vi "HX_Water-Props.vi"(8 "error in (no error)":errorcluster, 11 "Water Avg (°F)":dbl) -> (0 "error out":errorcluster, 2 "mu (lbm/ft*s)":dbl, 3 "Cp (BTU/lbm°F)":dbl, 4 "Density (lbm/ft³)":dbl)   [LabVIEW 2012]
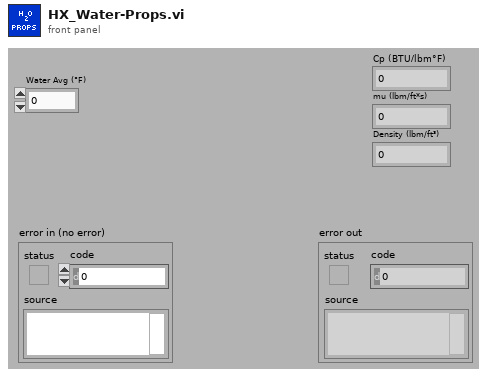
[diagram p1: front panel]
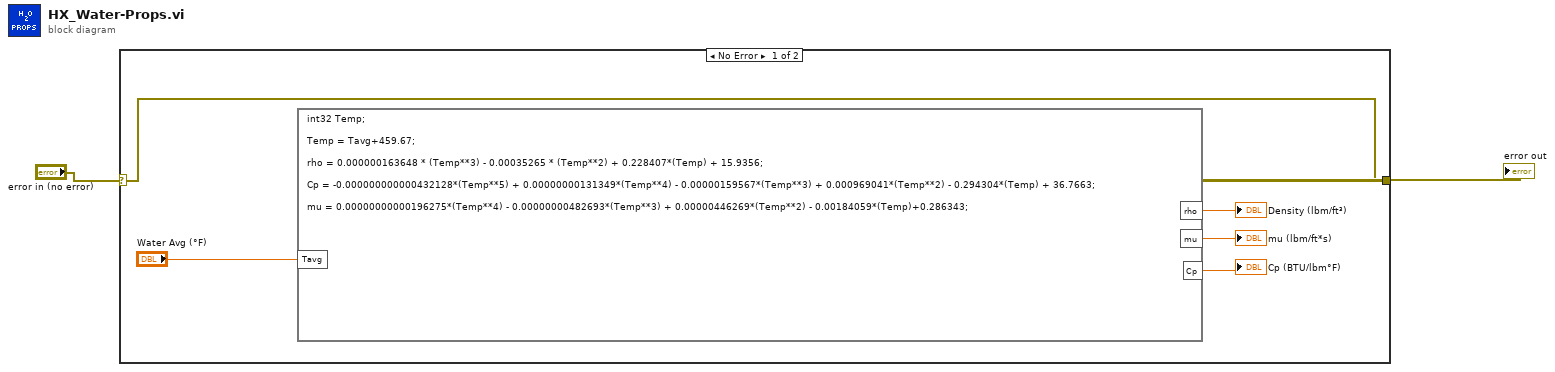
[diagram p0: block diagram]
diagram:
  n1 = case shown="No Error" "error in (no error)" {
    selector: "error in (no error)" -> [w3 w8]
    tunnel: [w3 w8] -> w1
    frame No Error {
      n2 = formula code="int32 Temp;\n \nTemp = Tavg+459.67;\n\nrho = 0.000000163648 * (Temp**3) - 0.00035265 * (Temp**2) + 0.228407*(Temp) + 15.9356;\n\nCp = -0.000000000000432128*(Temp**5) + 0.00000000131349*(Temp**4) - 0.00000159567*(Temp**3) + 0.000969041*(Temp**2) - 0.294304*(Temp) + 36.7663;\n\nmu = 0.00000000000196275*(Temp**4) - 0.00000000482693*(Temp**3) + 0.00000446269*(Temp**2) - 0.00184059*(Temp)+0.286343;"("Tavg"="Water Avg (°F)") -> ("rho"=→"Density (lbm/ft³)":dbl, "Cp"=→"Cp (BTU/lbm°F)":dbl, "mu"=→"mu (lbm/ft*s)":dbl)
    }
    frame Error {
    }
  }
  "error out" <- w1
